vi "Write.vi"(8 "error in (no error)":errorcluster, 10 "Write":sgl, 11 "Int_Single Float in":refnum<class "Int_Single Float.lvclass">) -> (0 "error out":errorcluster, 3 "Int_Single Float out":refnum<class "Int_Single Float.lvclass">)   [LabVIEW 2021, in "Int_Single Float.lvclass"]
uses:
  Int_Single Float.lvclass
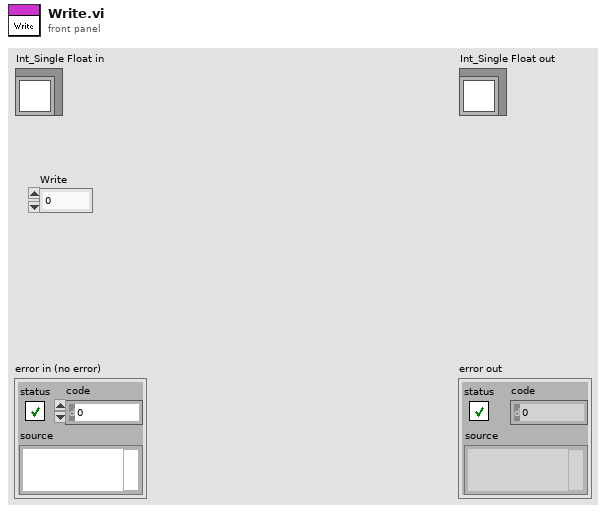
[diagram p1: front panel]
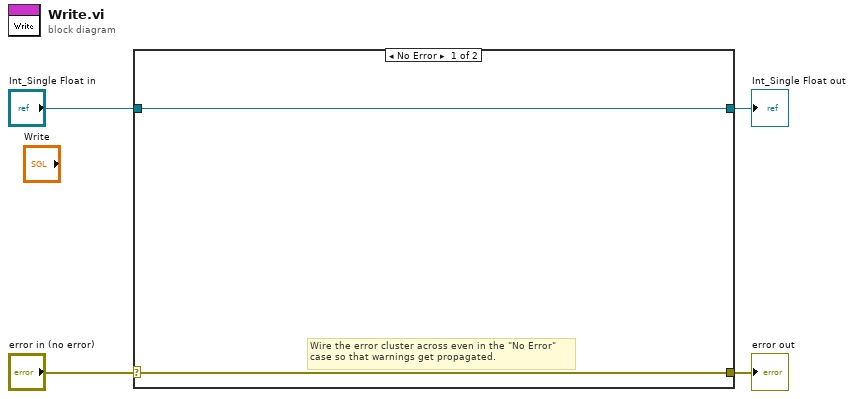
[diagram p0: block diagram]
diagram:
  n1 = case shown="No Error" "error in (no error)" {
    selector: "error in (no error)" -> [w5 w8]
    tunnel: [w5 w8] -> w3
    tunnel: [w6 w7] -> w1
    tunnel: "Int_Single Float in" -> [w6 w7]
    frame No Error {
      # "Wire the error cluster across even in the \"No Error\"\ncase so that warnings get propagated."
    }
    frame Error {
    }
  }
  "error out" <- w3
  "Int_Single Float out" <- w1
